vi "BUILD_ARRAYCONCATEVALUESSTOREIN_ARRAY.vi"() -> ()   [LabVIEW 2020]
uses:
  <vilib>/Utility/file.llb/Write Delimited Spreadsheet (string).vi
  <vilib>/Utility/file.llb/Write Delimited Spreadsheet (DBL).vi
panel:
  in  "Tab Control":enum32{"Page 1"}(tab)
  out "status":string
  out "completed":bool
  in  "file path (dialog if empty) excel file":path
  in  "file path (use dialog) for text file":path
  in  "file path (use dialog)":path
  out "appended array":dbl[][](array[numeric])
  out "error out":errorcluster
  in  "?":bool
  in  "stop":bool
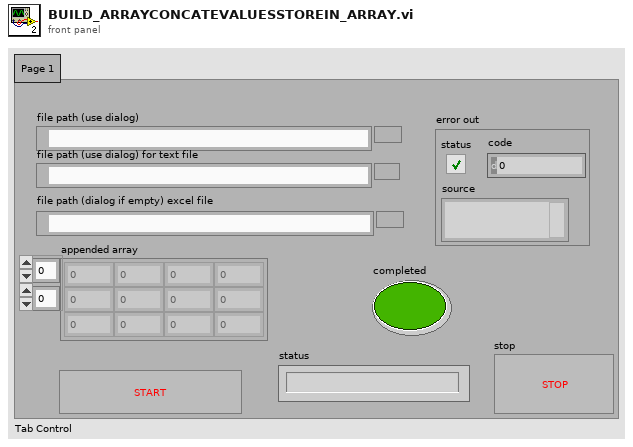
[diagram p1: front panel]
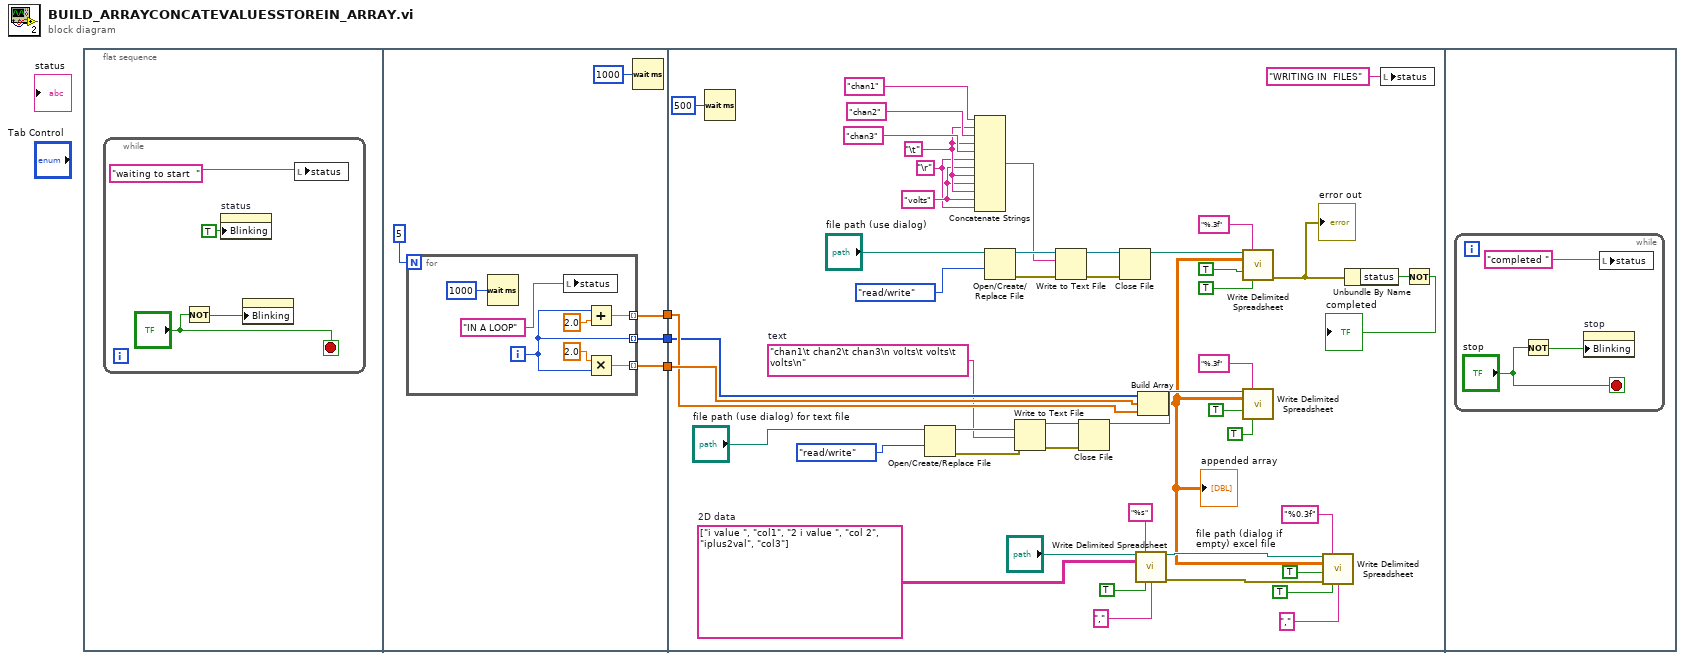
[diagram p0: block diagram]
diagram:
  n1 = flat-sequence {
    tunnel: [w10] -> w3
    tunnel: [w9] -> w2
    tunnel: [w11] -> w1
    tunnel: w3 -> [w58]
    tunnel: w2 -> [w57]
    tunnel: w1 -> [w49]
    frame #0 {
      n2 = while {
        stop <- "?" stop-if-true
        n3 = Not(x="?") -> (.not. x?=w7:bool)
        n4 = property on="status" class="Str"("Blinking"=TRUE) -> ()  [unwired: 2 in, 2 out]
        n5 = property class="Bool"("Blinking"=w7) -> ()  [unwired: 2 in, 2 out]
        n6 = local write "status"("waiting to start  " ("status")) -> ()
      }
    }
    frame #1 {
      n7 = for {
        N: 5 -> [_]
        tunnel: [w15] -> w11 mode=indexing
        tunnel: [w17] -> w10 mode=indexing
        tunnel: [w14] -> w9 mode=indexing
        i -> [w15]
        n8 = Wait (ms)(milliseconds to wait=u32 1000) -> ()  [unwired: 1 out]
        n9 = local write "status"("IN A LOOP" ("status")) -> ()
        n10 = Add(x=w15, y=2.0) -> (x+y=w14:dbl)
        n11 = Multiply(x=2.0, y=w15) -> (x*y=w17:dbl)
      }
      n12 = Wait (ms)(milliseconds to wait=u32 1000) -> ()  [unwired: 1 out]
    }
    frame #2 {
      w30 = "volts"
      w29 = "\r"
      w31 = "\t"
      w48 = "chan1\t chan2\t chan3\n volts\t volts\t volts\n"  # text
      w55 = string[][] [["i value ", "col1"], ["2 i value ", "col 2"], ["iplus2val", "col3"]]  # 2D data
      n13 = Wait (ms)(milliseconds to wait=u32 500) -> ()  [unwired: 1 out]
      n14 = Open/Create/Replace File(file path (use dialog)="file path (use dialog) for text file", access (0:read/write)=enum16{"read/write", "read-only", "write-only"}."read/write") -> (refnum out=w62:refnum<file>, error out=w61:errorcluster)  [unwired: 4 in, 1 out]
      n15 = Concatenate Strings("chan1" ("string"), w31, "chan2" ("string"), w31, "chan3" ("string"), w29, w30, w31, w30, w31, w30, w29) -> (w35:string)
      n16 = Open/Create/Replace File(file path (use dialog)="file path (use dialog)", access (0:read/write)=enum16{"read/write", "read-only", "write-only"}."read/write") -> (refnum out=w39:refnum<file>, error out=w40:errorcluster)  [unwired: 4 in, 1 out]
      n17 = Write to Text File(file (use dialog)=w62, text=w48, error in=w61) -> (refnum out=w60:refnum<file>, error out=w59:errorcluster)  [unwired: 1 in, 1 out]
      n18 = Write to Text File(file (use dialog)=w39, text=w35, error in=w40) -> (refnum out=w28:refnum<file>, error out=w41:errorcluster)  [unwired: 1 in, 1 out]
      n19 = Close File(refnum=w60, error in=w59) -> (path=w46:path)  [unwired: 1 out]
      n20 = Close File(refnum=w28, error in=w41) -> (path=w27:path)  [unwired: 1 out]
      n21 = call-poly <vilib>:"Write Delimited Spreadsheet.vi"("file path (dialog if empty)"="file path (dialog if empty) excel file", "format (%s)"="%s", "2D data"=w55, "transpose? (no:F)"=TRUE, "delimiter (\\t)"="," ("delimiter (\\t)")) -> ("new file path (Not A Path if cancelled)"=w52:path, "error out"=w51:errorcluster)  [unwired: 9 in]
      n22 = Build Array(w49, w58, w57) -> (w26:dbl[][])
      "appended array" <- w26
      n23 = call-poly <vilib>:"Write Delimited Spreadsheet.vi"("file path (dialog if empty)"=w27, "format (%.3f)"="%.3f", "2D data"=w26, "append to file? (new file:F)"=TRUE, "transpose? (no:F)"=TRUE) -> ("error out"=w25:errorcluster)  [unwired: 9 in, 1 out]
      "error out" <- w25
      n24 = call-poly <vilib>:"Write Delimited Spreadsheet.vi"("file path (dialog if empty)"=w46, "format (%.3f)"="%.3f", "2D data"=w26, "append to file? (new file:F)"=TRUE, "transpose? (no:F)"=TRUE) -> ()  [unwired: 9 in, 2 out]
      n25 = call-poly <vilib>:"Write Delimited Spreadsheet.vi"("file path (dialog if empty)"=w52, "format (%.3f)"="%0.3f", "2D data"=w26, "append to file? (new file:F)"=TRUE, "error in (no error)"=w51, "transpose? (no:F)"=TRUE, "delimiter (\\t)"="," ("delimiter (\\t)")) -> ()  [unwired: 7 in, 2 out]
      n26 = Unbundle By Name(w25) -> ("status"=w24:bool)
      n27 = local write "status"("WRITING IN  FILES" ("status")) -> ()
      n28 = Not(x=w24) -> (.not. x?=→"completed":bool)
    }
    frame #3 {
      n29 = while {
        stop <- "stop" stop-if-true
        n30 = Not(x="stop") -> (.not. x?=w69:bool)
        n31 = property on="stop" class="Bool"("Blinking"=w69) -> ()  [unwired: 2 in, 2 out]
        n32 = local write "status"("completed " ("status")) -> ()
      }
    }
  }
